vi "CRYDataView Function LIB.vi"(7 "sAction":string, 8 "nData":i32, 9 "sData":string, 10 "sOption":string, 11 "cBootVIEW":T1) -> (0 "nData_Out":i32, 1 "sData_Out":string, 3 "cView_Out":T2)   [LabVIEW 2013]
uses:
  CRYView Global.vi
  CRYNew View Global.vi
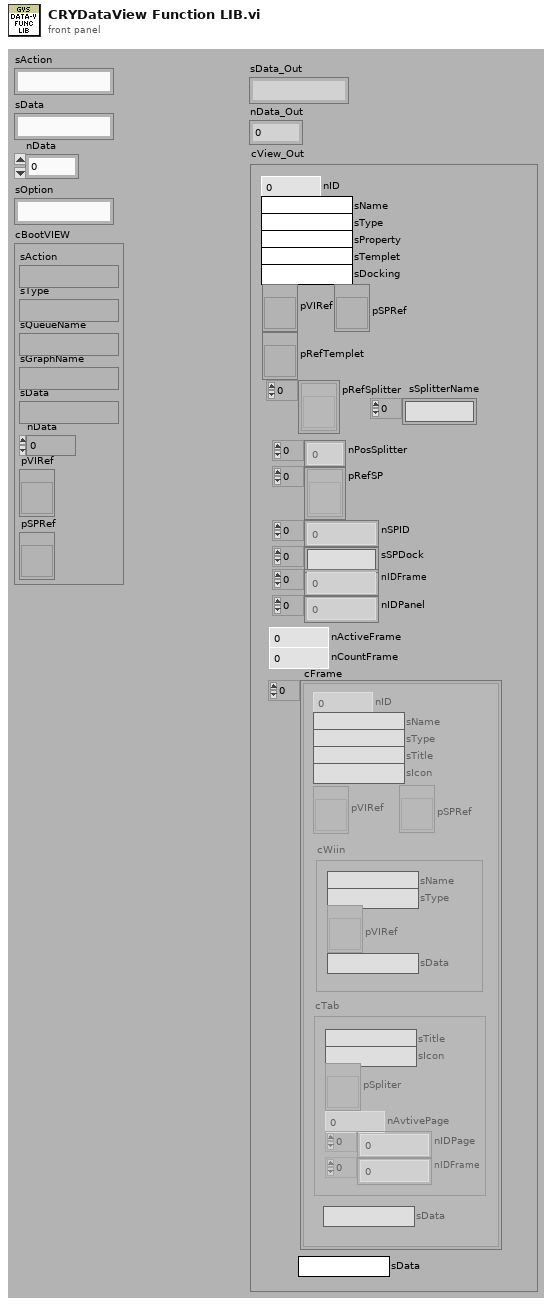
[diagram p1: front panel]
types:
  T1 = cluster{"sAction":string, "sType":string, "sQueueName":string, "sGraphName":string, "sData":string, "nData":i32, "pVIRef":refnum<vi>, "pSPRef":refnum<vi>}
  T2 = cluster{"nID":i32, "sName":string, "sType":string, "sProperty":string, "sTemplet":string, "sDocking":string, "pVIRef":refnum<vi>, "pSPRef":refnum<vi>, "pRefTemplet":refnum<vi>, "pRefSplitter":refnum<vi>[], "nPosSplitter":i32[], "pRefSP":refnum<vi>[], "nSPID":i32[], "sSPDock":string[], "nIDFrame":i32[], "nIDPanel":i32[], "nActiveFrame":i32, "nCountFrame":i32, "cFrame":cluster{"nID":i32, "sName":string, "sType":string, "sTitle":string, "sIcon":string, "pVIRef":refnum<vi>, "pSPRef":refnum<vi>, "cWiin":cluster{"sName":string, "sType":string, "pVIRef":refnum<vi>, "sData":string}, "cTab":cluster{"sTitle":string, "sIcon":string, "pSpliter":refnum<vi>, "nAvtivePage":i32, "nIDPage":i32[], "nIDFrame":i32[]}, "sData":string}[], "sData":string, "sSplitterName":string[]}
  T3 = cluster{"nID":i32, "sTiltle":string, "pVI":refnum<vi>, "pSP":refnum<vi>, "pTab":refnum<vi>, "pSPT":refnum<vi>, "nWinType":i32, "sIcon":string}
  T4 = cluster{"nID":i32, "sName":string, "sType":string, "sProperty":string, "sTemplet":string, "sDocking":string, "pVIRef":refnum<vi>, "pSPRef":refnum<vi>, "pRefTemplet":refnum<vi>, "pRefSplitter":refnum<vi>[], "nPosSplitter":i32[], "pRefSP":refnum<vi>[], "nSPID":i32[], "sSPDock":string[], "nIDFrame":i32[], "nIDPanel":i32[], "nActiveFrame":i32, "nCountFrame":i32, "cFrame":cluster{"nID":i32, "sName":string, "sType":string, "sTitle":string, "sIcon":string, "pVIRef":refnum<vi>, "pSPRef":refnum<vi>, "cWin":cluster{"sName":string, "sType":string, "pVIRef":refnum<vi>, "sData":string}, "cTab":cluster{"sTitle":string, "sIcon":string, "pSpliter":refnum<vi>, "nAvtivePage":i32, "nIDPage":i32[], "nIDFrame":i32[]}, "sData":string}[], "sData":string, "sSplitterName":string[]}
  T5 = typedef "Graph Main Info Cluster.ctl" = cluster{"Selected_BarIdx":i32, "Selected_PanelIdx":i32, "Graph Main VIRef":refnum<vi>, "ToolBarClick":bool, "Spliter Ref Array":refnum<vi>[], "Panel Ref Array":refnum<vi>[], "Spliter_matrix":i32[][], "Panel_matrix":i32[][], "child_spliterIdx_matrix":i32[][], "split_pos_matrix":i32[][], "Title State":bool, "sQueueName":string, "Frame nID":i32, "Graph VIRef Array":cluster{"Graph VIRef":refnum<vi>, "Panel Idx":i32, "Frame VIRef":refnum<vi>, "Icon Ring":i32, "Graph Type":string}[], "View Type":string}
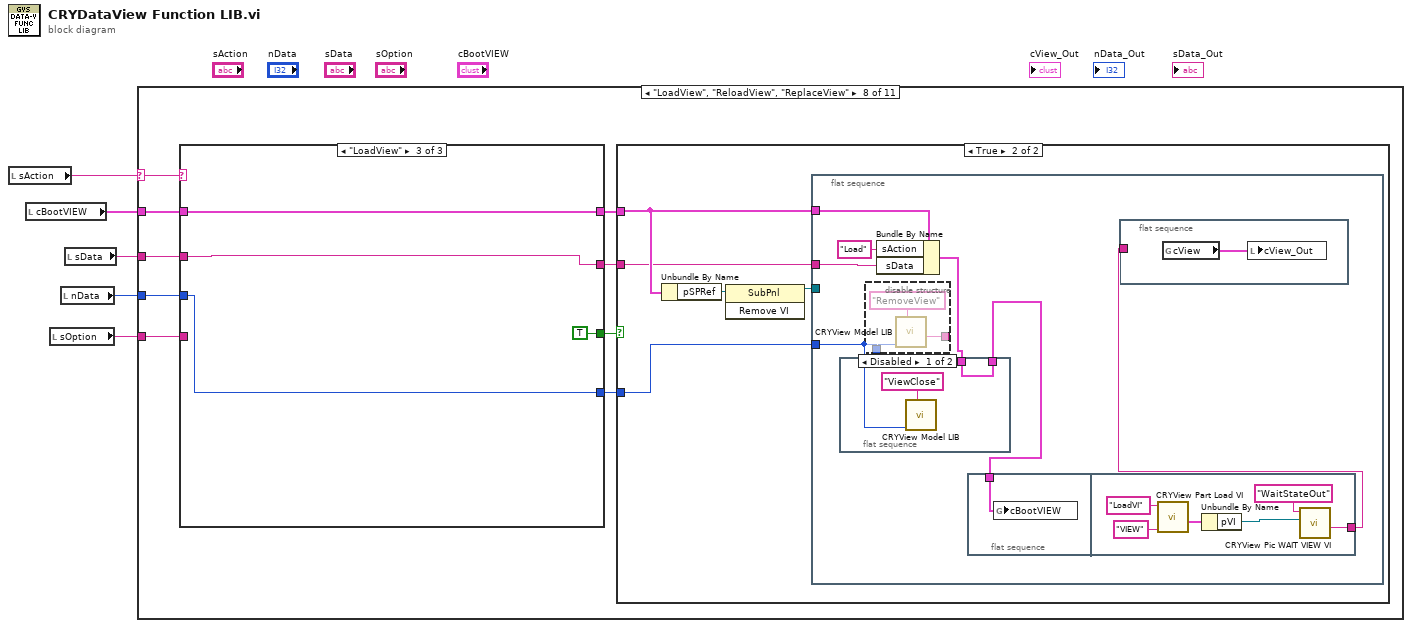
[diagram p0: block diagram]
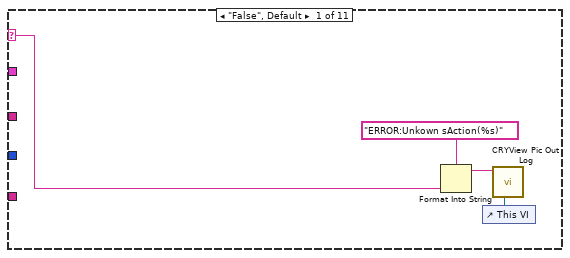
[diagram p2: hidden frame]
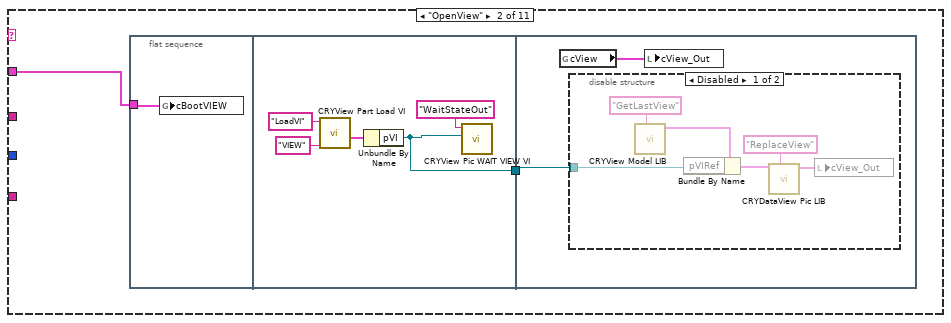
[diagram p3: hidden frame]
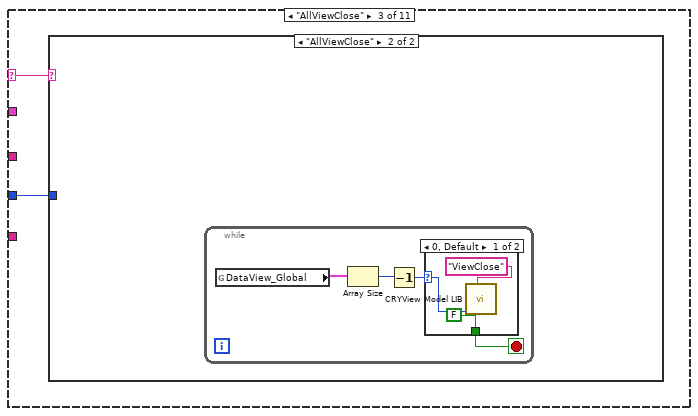
[diagram p5: hidden frame]
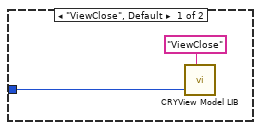
[diagram p6: hidden frame]
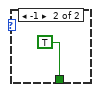
[diagram p7: hidden frame]
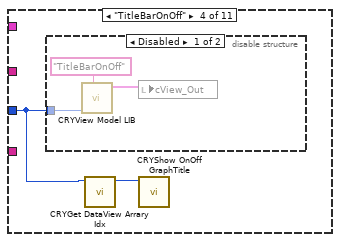
[diagram p8: hidden frame]
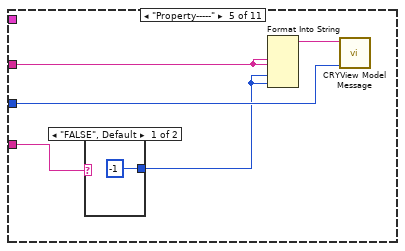
[diagram p10: hidden frame]
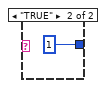
[diagram p11: hidden frame]
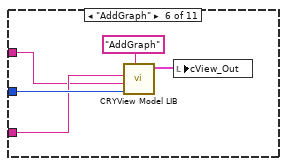
[diagram p12: hidden frame]
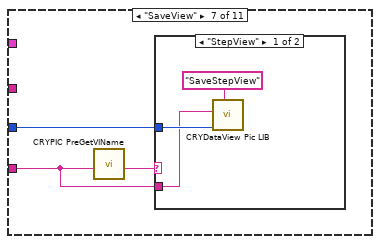
[diagram p13: hidden frame]
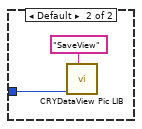
[diagram p14: hidden frame]
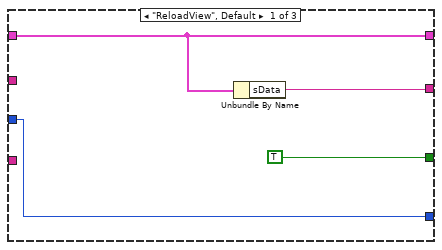
[diagram p17: hidden frame]
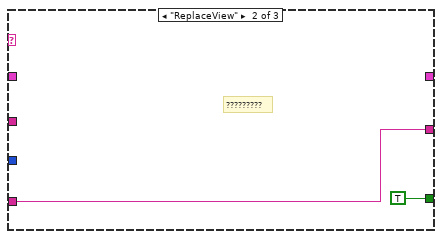
[diagram p18: hidden frame]
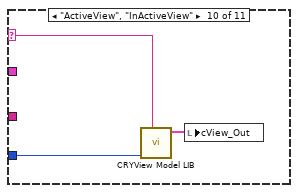
[diagram p20: hidden frame]
diagram:
  n1 = local read "sAction"() -> (w1:string)
  n2 = local read "cBootVIEW"() -> (w2:T1)
  n3 = local read "sOption"() -> (w3:string)
  n4 = local read "nData"() -> (w4:i32)
  n5 = local read "sData"() -> (w5:string)
  n6 = case shown="\"LoadView\", \"ReloadView\", \"ReplaceView\"" w1 {
    selector: w1 -> [w7 _ w26 _ _ _ _ w68 _ w109 _]
    tunnel: w5 -> [_ _ _ _ w45 w51 _ w70 _ _ _]
    tunnel: w4 -> [_ _ w27 w39 w46 w53 w57 w71 _ w108 w113]
    tunnel: w3 -> [_ _ _ _ w44 w52 w55 w63 _ _ _]
    tunnel: w2 -> [_ w10 _ _ _ _ _ w69 _ _ _]
    frame "False", Default {
      n7 = Format Into String(format string="ERROR:Unkown sAction(%s)", w7) -> (resulting string=w6:string)  [unwired: 2 in, 1 out]
      n8 = control-ref of="This VI"() -> (w9:refnum<vi>)
      n9 = call "CRYView Pic Out Log.vi"("vi reference"=w9, "sData"=w6) -> ()  [unwired: 10 in]
    }
    frame "OpenView" {
      n10 = flat-sequence {
        tunnel: w10 -> [w12]
        tunnel: [w14] -> w11
        tunnel: w11 -> [w19]
        frame #0 {
          n11 = global write "CRYView Global.vi" "cBootVIEW"(w12) -> ()
        }
        frame #1 {
          n12 = call "CRYView Part Load VI.vi"("sData"="VIEW", "sAction"="LoadVI") -> ("tWindow_Out"=w17:T3)  [unwired: 9 in]
          n13 = Unbundle By Name(w17) -> ("pVI"=w14:refnum<vi>)
          n14 = call "CRYView Pic WAIT VIEW VI.vi"("vi reference"=w14, "sAction"="WaitStateOut") -> ()  [unwired: 9 in, 1 out]
        }
        frame #2 {
          n15 = global read "CRYView Global.vi" "cView"() -> (w18:T4)
          n16 = disable-structure shown="Disabled" {
            disable-tunnel: w19 -> [w25 _]
            frame Disabled {
              n17 = call "CRYView Model LIB.vi"("sAction"="GetLastView") -> ("cView_Out"=w23:T2)  [unwired: 8 in, 2 out]
              n18 = Bundle By Name(cluster=w23, "pVIRef"=w25) -> (w22:T2)
              n19 = call "CRYDataView Pic LIB.vi"("sAction"="ReplaceView", "cView"=w22) -> ("cView_Out"=w20:T2)  [unwired: 7 in, 2 out]
              n20 = local write "cView_Out"(w20) -> ()
            }
            frame Enabled {
            }
          }
          n21 = local write "cView_Out"(w18) -> ()
        }
      }
    }
    frame "AllViewClose" {
      n22 = case shown="\"AllViewClose\"" w26 {
        tunnel: w27 -> [w28 _]
        frame "ViewClose", Default {
          n23 = call "CRYView Model LIB.vi"("sAction"="ViewClose", "nData"=w28) -> ()  [unwired: 7 in, 3 out]
        }
        frame "AllViewClose" {
          n24 = while {
            stop <- w30 stop-if-true
            n25 = global read "CRYNew View Global.vi" "DataView_Global"() -> (w33:T5[])
            n26 = Array Size(array=w33) -> (size(s)=w32:i32)
            n27 = Decrement(x=w32) -> (x-1=w31:i32)
            n28 = case shown="0, Default" w31 {
              selector: w31 -> [w35 _]
              tunnel: [FALSE TRUE] -> w30
              frame 0, Default {
                n29 = call "CRYView Model LIB.vi"("sAction"="ViewClose", "nData"=w35) -> ()  [unwired: 7 in, 3 out]
              }
              frame -1 {
              }
            }
          }
        }
      }
    }
    frame "TitleBarOnOff" {
      n30 = disable-structure shown="Disabled" {
        disable-tunnel: w39 -> [w41 _]
        frame Disabled {
          n31 = call "CRYView Model LIB.vi"("sAction"="TitleBarOnOff", "nData"=w41) -> ("cView_Out"=w40:T2)  [unwired: 7 in, 2 out]
          n32 = local write "cView_Out"(w40) -> ()
        }
        frame Enabled {
        }
      }
      n33 = call "CRYGet DataView Arrary Idx.vi"("DataView Idx In"=w39) -> ("DataView Arrary Idx out"=w38:i32)  [unwired: 10 in]
      n34 = call "CRYShow OnOff GraphTitle.vi"("DataView Array Idx"=w38) -> ()  [unwired: 11 in]
    }
    frame "Property-----" {
      n35 = case shown="\"FALSE\", Default" w44 {
        tunnel: [-1 1] -> w43
        frame "FALSE", Default {
        }
        frame "TRUE" {
        }
      }
      n36 = Format Into String(w45, w45, w43, w43) -> (resulting string=w47:string)  [unwired: 3 in, 1 out]
      n37 = call "CRYView Model Message.vi"("nData"=w46, "sMsgData"=w47) -> ()  [unwired: 7 in, 3 out]
    }
    frame "AddGraph" {
      n38 = call "CRYView Model LIB.vi"("sAction"="AddGraph", "nData"=w53, "sData"=w51, "sOption"=w52) -> ("cView_Out"=w50:T2)  [unwired: 5 in, 2 out]
      n39 = local write "cView_Out"(w50) -> ()
    }
    frame "SaveView" {
      n40 = call "CRYPIC PreGetVIName.vi"("sVIName"=w55) -> ("sVIName_Out"=w56:string)  [unwired: 9 in, 1 out]
      n41 = case shown="\"StepView\"" w56 {
        tunnel: w57 -> [w60 w62]
        tunnel: w55 -> [w58 _]
        frame "StepView" {
          n42 = call "CRYDataView Pic LIB.vi"("sAction"="SaveStepView", "nData"=w60, "sOption"=w58) -> ()  [unwired: 6 in, 3 out]
        }
        frame Default {
          n43 = call "CRYDataView Pic LIB.vi"("sAction"="SaveView", "nData"=w62) -> ()  [unwired: 7 in, 3 out]
        }
      }
    }
    frame "LoadView", "ReloadView", "ReplaceView" {
      n44 = case shown="\"LoadView\"" w68 {
        tunnel: w71 -> [w101 _ w106]
        tunnel: w70 -> [_ _ w105]
        tunnel: w69 -> [w100 _ w107]
        tunnel: [w100 _ w107] -> w67
        tunnel: [w101 _ w106] -> w66
        tunnel: [TRUE TRUE TRUE] -> w65
        tunnel: [w98 w102 w105] -> w64
        tunnel: w63 -> [_ w102 _]
        frame "ReloadView", Default {
          n45 = Unbundle By Name(w100) -> ("sData"=w98:string)
        }
        frame "ReplaceView" {
          # "?????????"
        }
        frame "LoadView" {
        }
      }
      n46 = case shown="True" w65 {
        tunnel: w67 -> [_ w74]
        tunnel: w66 -> [_ w73]
        tunnel: w64 -> [_ w72]
        frame False {
        }
        frame True {
          n47 = Unbundle By Name(w74) -> ("pSPRef"=w76:refnum<vi>)
          n48 = invoke class="SubPnl" method="Remove VI"(reference=w76) -> (reference out=w75:refnum<vi>)  [unwired: 2 in, 2 out]
          n49 = flat-sequence {
            tunnel: w72 -> [w82]
            tunnel: w73 -> [w80]
            tunnel: w74 -> [w81]
            tunnel: w75 -> [_]
            frame #0 {
              n50 = flat-sequence {
                tunnel: w80 -> [w93]
                tunnel: w79 -> [w92]
                tunnel: [w92] -> w78
                frame #0 {
                  n51 = call "CRYView Model LIB.vi"("sAction"="ViewClose", "nData"=w93) -> ()  [unwired: 7 in, 3 out]
                }
              }
              n52 = disable-structure shown="Disabled" {
                disable-tunnel: [w96 _] -> _
                disable-tunnel: w80 -> [w95 _]
                frame Disabled {
                  n53 = call "CRYView Model LIB.vi"("sAction"="RemoveView", "nData"=w95) -> ("sData_Out"=w96:string)  [unwired: 7 in, 2 out]
                }
                frame Enabled {
                }
              }
              n54 = Bundle By Name(cluster=w81, "sAction"="Load", "sData"=w82) -> (w79:T1)
              n55 = flat-sequence {
                tunnel: w78 -> [w85]
                tunnel: [w86] -> w77
                frame #0 {
                  n56 = global write "CRYView Global.vi" "cBootVIEW"(w85) -> ()
                }
                frame #1 {
                  n57 = call "CRYView Part Load VI.vi"("sData"="VIEW", "sAction"="LoadVI") -> ("tWindow_Out"=w91:T3)  [unwired: 9 in]
                  n58 = Unbundle By Name(w91) -> ("pVI"=w88:refnum<vi>)
                  n59 = call "CRYView Pic WAIT VIEW VI.vi"("vi reference"=w88, "sAction"="WaitStateOut") -> ("sData_Out"=w86:string)  [unwired: 9 in]
                }
              }
              n60 = flat-sequence {
                tunnel: w77 -> [_]
                frame #0 {
                  n61 = global read "CRYView Global.vi" "cView"() -> (w84:T4)
                  n62 = local write "cView_Out"(w84) -> ()
                }
              }
            }
          }
        }
      }
    }
    frame "CloseViewData" {
    }
    frame "ActiveView", "InActiveView" {
      n63 = call "CRYView Model LIB.vi"("sAction"=w109, "nData"=w108) -> ("cView_Out"=w110:T2)  [unwired: 7 in, 2 out]
      n64 = local write "cView_Out"(w110) -> ()
    }
    frame "GetViewByID" {
      n65 = call "CRYView Model LIB.vi"("sAction"="GetViewByID", "nData"=w113) -> ("cView_Out"=w112:T2)  [unwired: 7 in, 2 out]
      n66 = Unbundle By Name(w112) -> ("nID"=w111:i32)
      n67 = local write "cView_Out"(w112) -> ()
      n68 = local write "nData_Out"(w111) -> ()
    }
  }
